vi "Load Sub Panel.vi"(8 "error in (no error)":errorcluster, 10 "sub panel ref":refnum<vi>, 11 "Logger Normal in":refnum<class "Logger Normal.lvclass">) -> (0 "error out":errorcluster, 3 "Logger Normal out":refnum<class "Logger Normal.lvclass">)   [LabVIEW 2020, in "Logger Normal.lvlib" / "Logger Normal.lvclass"]
uses:
  Logger Normal.lvclass
  Logger/Logger Messages/Insert VI Msg/Insert VI Msg.lvclass
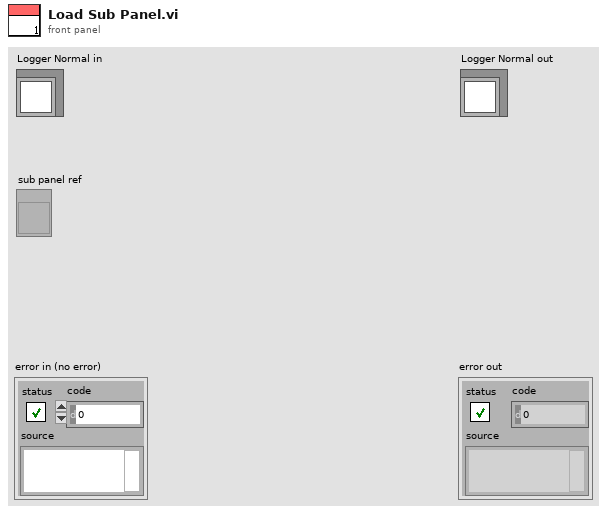
[diagram p1: front panel]
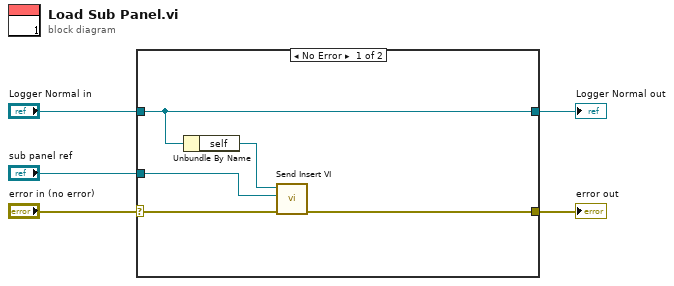
[diagram p0: block diagram]
diagram:
  n1 = case shown="No Error" "error in (no error)" {
    selector: "error in (no error)" -> [w9 w11]
    tunnel: "sub panel ref" -> [w6 _]
    tunnel: "Logger Normal in" -> [w10 w12]
    tunnel: [w10 w12] -> w2
    tunnel: [w8 w11] -> w1
    frame No Error {
      n2 = Unbundle By Name(w10) -> ("self"=w7:refnum<class "Message Enqueuer.lvclass">)
      n3 = call "Send Insert VI.vi"("error in (no error)"=w9, "sub panel"=w6, "Message Enqueuer"=w7) -> ("error out"=w8:errorcluster)  [unwired: 7 in, 1 out]
    }
    frame Error {
    }
  }
  "error out" <- w1
  "Logger Normal out" <- w2
